vi "Implement Constructor.vi"(8 "error in (no error)":errorcluster, 10 "Constructor Path":path, 11 "Mock Class Generator in":refnum<class "Mock Class Generator.lvclass">) -> (0 "error out":errorcluster, 3 "Mock Class Generator":refnum<class "Mock Class Generator.lvclass">)   [LabVIEW 2020, in "Mock Class Generator.lvclass"]
uses:
  Mock Class Generator.lvclass
  <vilib>/Utility/traverseref.llb/TRef TravTarget.ctl
  Mock Class Generator.lvclass/Mock Class Generator.ctl
  <vilib>/Utility/traverseref.llb/VI Scripting - Traverse.lvlib
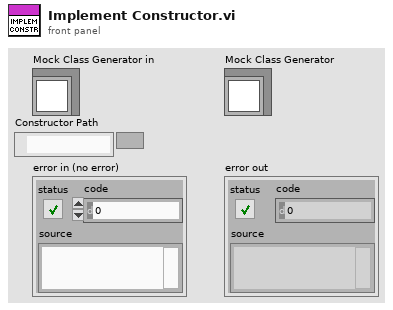
[diagram p1: front panel]
types:
  T1 = typedef "TRef TravTarget.ctl" = enum16{"FP", "BD", "Other"}
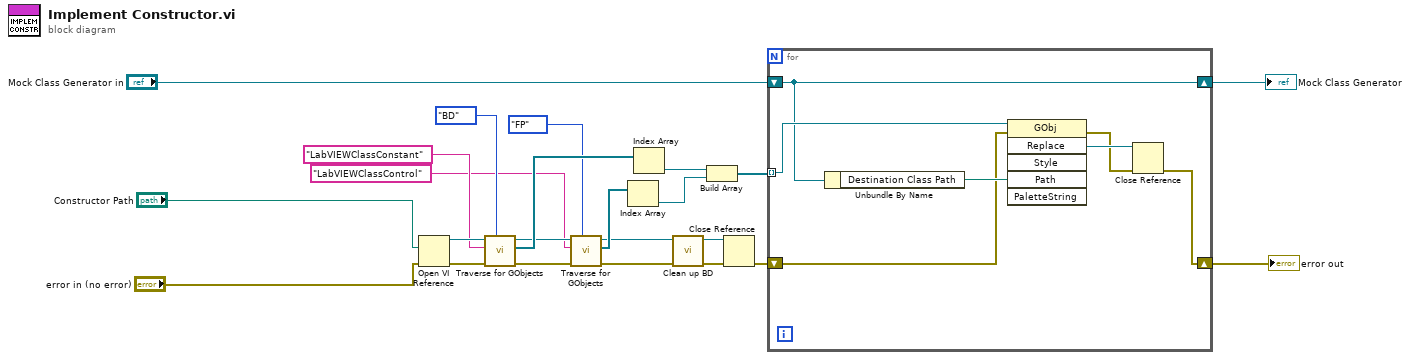
[diagram p0: block diagram]
diagram:
  n1 = Open VI Reference(vi path="Constructor Path", error in (no error)="error in (no error)") -> (vi reference=w20:refnum<vi>, error out=w23:errorcluster)  [unwired: 4 in]
  n2 = call <vilib>:"Traverse for GObjects.vi"("Traverse Target"=TRef_TravTarget."BD", "error in (no error)"=w23, "Class Name"="LabVIEWClassConstant", "VI Refnum"=w20) -> ("error out"=w11:errorcluster, "References"=w17:refnum<vi>[], "dup VI Refnum"=w12:refnum<vi>)  [unwired: 4 in, 1 out]
  n3 = call <vilib>:"Traverse for GObjects.vi"("Traverse Target"=TRef_TravTarget."FP", "error in (no error)"=w11, "Class Name"="LabVIEWClassControl", "VI Refnum"=w12) -> ("error out"=w6:errorcluster, "References"=w8:refnum<vi>[], "dup VI Refnum"=w3:refnum<vi>)  [unwired: 4 in, 1 out]
  n4 = Index Array(array=w8) -> (element=w7:refnum<vi>)  [unwired: 1 in]
  n5 = Index Array(array=w17) -> (element=w16:refnum<vi>)  [unwired: 1 in]
  n6 = call "Clean up BD.vi"("error in (no error)"=w6, "VI in"=w3) -> ("error out"=w4:errorcluster, "VI out"=w1:refnum<vi>)  [unwired: 8 in]
  n7 = Build Array(w16, w7) -> (w14:refnum<vi>[])
  n8 = Close Reference(reference=w1, error in (no error)=w4) -> (error out=w2:errorcluster)
  n9 = for {
    tunnel: w14 -> [w29] mode=indexing
    shift-right: [w24] -> w5
    shift-left: w2 -> [w28]
    shift-right: [w26] -> w13
    shift-left: "Mock Class Generator in" -> [w26]
    n10 = Unbundle By Name(w26) -> ("Destination Class Path"=w30:path)
    n11 = invoke class="GObj" method="Replace"(reference=w29, error in=w28, "Path"=w30) -> (error out=w25:errorcluster, "Replace"=w27:refnum<vi>)  [unwired: 3 in, 4 out]
    n12 = Close Reference(reference=w27, error in (no error)=w25) -> (error out=w24:errorcluster)
  }
  "Mock Class Generator" <- w13
  "error out" <- w5
